vi "range_check.vi"(7 "data value":dbl, 11 "config file key":string) -> (1 "color out":u32, 3 "error?":bool)   [LabVIEW 2017]
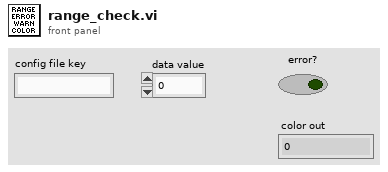
[diagram p1: front panel]
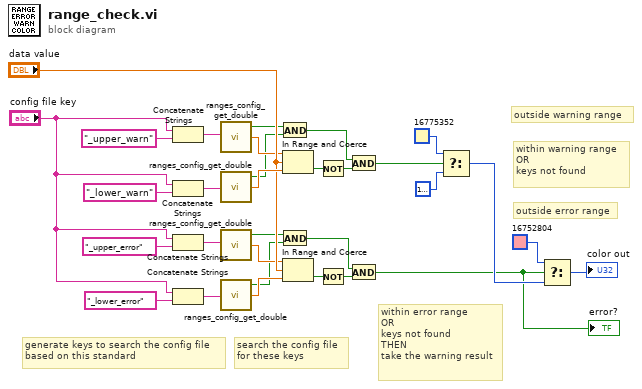
[diagram p0: block diagram]
diagram:
  # "search the config file\nfor these keys"
  # "generate keys to search the config file\nbased on this standard"
  # "outside error range"
  # "within error range\nOR\nkeys not found\nTHEN\ntake the warning result"
  # "within warning range\nOR\nkeys not found"
  # "outside warning range"
  n1 = Concatenate Strings("config file key", "_upper_warn" ("string")) -> (w28:string)
  n2 = Concatenate Strings("config file key", "_lower_warn" ("string")) -> (w25:string)
  n3 = Concatenate Strings("config file key", "_upper_error" ("string")) -> (w24:string)
  n4 = Concatenate Strings("config file key", "_lower_error" ("string")) -> (w21:string)
  n5 = call "ranges_config_get_double.vi"("key"=w28) -> ("value"=w29:dbl, "found?"=w17:bool)  [unwired: 3 in]
  n6 = call "ranges_config_get_double.vi"("key"=w25) -> ("value"=w31:dbl, "found?"=w16:bool)  [unwired: 3 in]
  n7 = call "ranges_config_get_double.vi"("key"=w24) -> ("value"=w19:dbl, "found?"=w15:bool)  [unwired: 3 in]
  n8 = call "ranges_config_get_double.vi"("key"=w21) -> ("value"=w18:dbl, "found?"=w14:bool)  [unwired: 3 in]
  n9 = And(x=w17, y=w16) -> (x .and. y?=w10:bool)
  n10 = And(x=w15, y=w14) -> (x .and. y?=w8:bool)
  n11 = In Range and Coerce(upper limit=w29, x="data value", lower limit=w31) -> (In Range?=w13:bool)  [unwired: 1 out]
  n12 = In Range and Coerce(upper limit=w19, x="data value", lower limit=w18) -> (In Range?=w12:bool)  [unwired: 1 out]
  n13 = Not(x=w13) -> (.not. x?=w11:bool)
  n14 = Not(x=w12) -> (.not. x?=w9:bool)
  n15 = And(x=w10, y=w11) -> (x .and. y?=w7:bool)
  n16 = And(x=w8, y=w9) -> (x .and. y?=w1:bool)
  "error?" <- w1
  n17 = Select(t=u32 16775352 ("Foreground Color"), s=w7, f=u32 16777238 ("Background Color")) -> (s? t:f=w3:u32)
  n18 = Select(t=u32 16752804 ("Foreground Color"), s=w1, f=w3) -> (s? t:f=→"color out":u32)
